vi "Read Instr XML File.vi"(0 "XML File Name":string, 5 "error in (no error)":errorcluster) -> (10 "Instr 1 Resource Str":string, 11 "Instr 4 Class Path":path, 12 "Instr 1 Class Path":path, 13 "Instr 4 Resource Str":string, 14 "Instr 2 Resource Str":string, 15 "Instr 2 Class Path":path, 16 "Instr 3 Resource Str":string, 17 "Instr 3 Class Path":path, 19 "error IO":errorcluster)   [LabVIEW 2010]
doc: "Reads an XML file with the DSSP module and hardware resource name information."
uses:
  <vilib>/Utility/xml.llb/Read From XML File(array).vi
panel:
  out "Instr 4 type":string
  out "Instr 3 type":string
  out "Instr 2 type":string
  out "Instr 1 type":string
  out "XML File Path Out":path
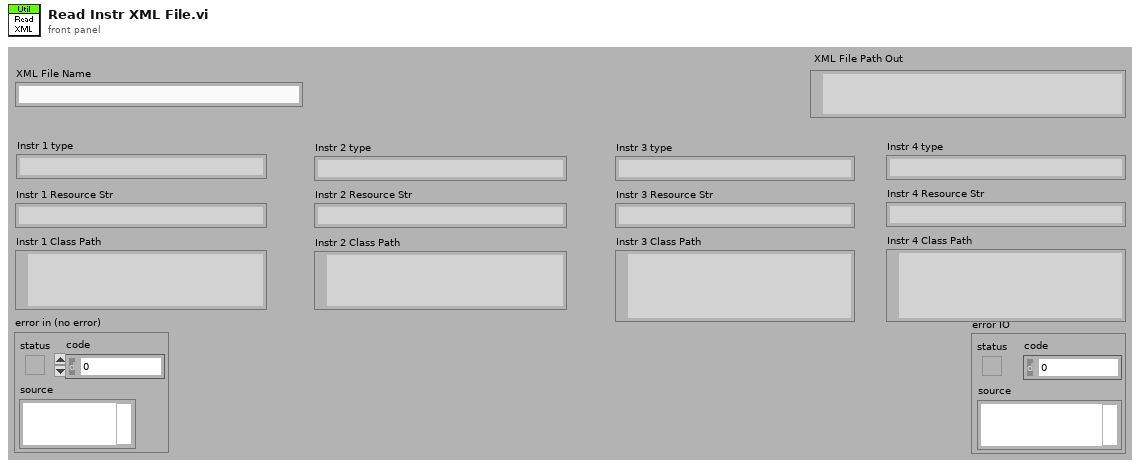
[diagram p1: front panel]
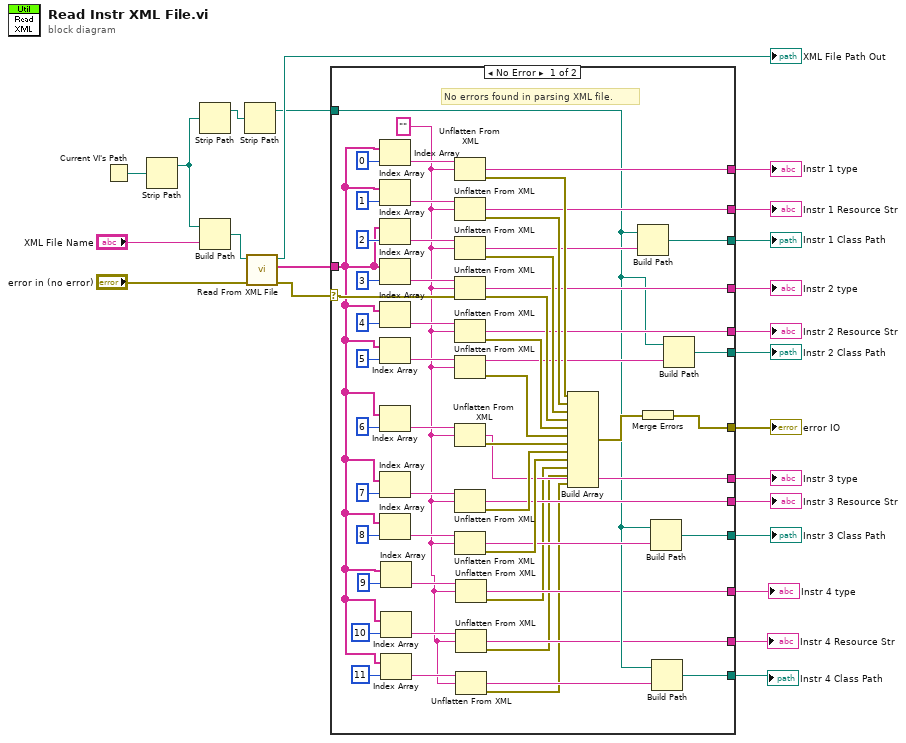
[diagram p0: block diagram]
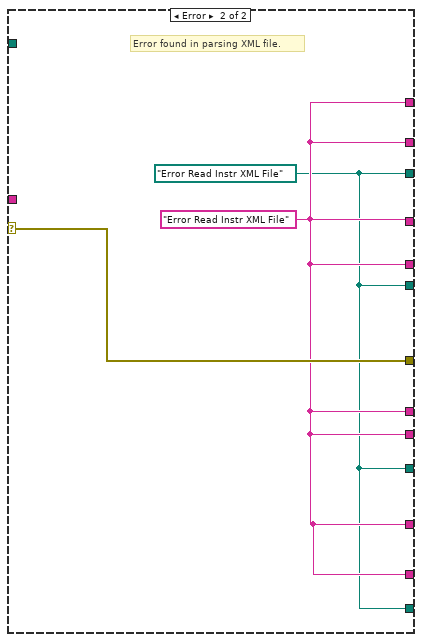
[diagram p2: hidden frame]
diagram:
  n1 = Current VI's Path() -> (path=w9:path)
  n2 = Strip Path(path=w9) -> (stripped path=w7:path)  [unwired: 1 out]
  n3 = Strip Path(path=w7) -> (stripped path=w5:path)  [unwired: 1 out]
  n4 = Build Path(base path=w7, name or relative path="XML File Name") -> (appended path=w8:path)
  n5 = Strip Path(path=w5) -> (stripped path=w4:path)  [unwired: 1 out]
  n6 = call-poly <vilib>:"Read From XML File.vi"("error in (no error)"="error in (no error)", "XML File Path"=w8) -> ("error out"=w21:errorcluster, "XML Elements"=w22:string[], "XML File Path(duplicate)"=→"XML File Path Out":path)  [unwired: 7 out]
  n7 = case shown="No Error" w21 {
    selector: w21 -> [w47 w84]
    tunnel: w22 -> [w36 _]
    tunnel: [w68 w84] -> w13
    tunnel: [w50 w83] -> w20
    tunnel: [w44 w82] -> w19
    tunnel: [w52 w83] -> w18
    tunnel: [w42 w82] -> w17
    tunnel: [w51 w83] -> w16
    tunnel: [w40 w82] -> w15
    tunnel: [w49 w83] -> w12
    tunnel: [w48 w83] -> w11
    tunnel: [w46 w83] -> w10
    tunnel: w4 -> [w31 _]
    tunnel: [w29 w82] -> w3
    tunnel: [w28 w83] -> w2
    tunnel: [w27 w83] -> w1
    frame No Error {
      w32 = ""
      # "No errors found in parsing XML file."
      n8 = Index Array(array=w36, index=0) -> (element=w77:string)
      n9 = Index Array(array=w36, index=1) -> (element=w76:string)
      n10 = Index Array(array=w36, index=2) -> (element=w75:string)
      n11 = Index Array(array=w36, index=3) -> (element=w74:string)
      n12 = Index Array(array=w36, index=4) -> (element=w62:string)
      n13 = Index Array(array=w36, index=5) -> (element=w61:string)
      n14 = Index Array(array=w36, index=6) -> (element=w60:string)
      n15 = Index Array(array=w36, index=7) -> (element=w59:string)
      n16 = Index Array(array=w36, index=8) -> (element=w58:string)
      n17 = Index Array(array=w36, index=9) -> (element=w33:string)
      n18 = Index Array(array=w36, index=10) -> (element=w35:string)
      n19 = Index Array(array=w36, index=11) -> (element=w34:string)
      n20 = Unflatten From XML(xml string=w77, type=w32) -> (value=w50:string, error out=w73:errorcluster)  [unwired: 1 in]
      n21 = Unflatten From XML(xml string=w76, type=w32) -> (value=w49:string, error out=w72:errorcluster)  [unwired: 1 in]
      n22 = Unflatten From XML(xml string=w75, type=w32) -> (value=w45:string, error out=w71:errorcluster)  [unwired: 1 in]
      n23 = Unflatten From XML(xml string=w74, type=w32, error in (no error)=w47) -> (value=w52:string, error out=w70:errorcluster)
      n24 = Unflatten From XML(xml string=w62, type=w32) -> (value=w48:string, error out=w57:errorcluster)  [unwired: 1 in]
      n25 = Unflatten From XML(xml string=w61, type=w32) -> (value=w41:string, error out=w56:errorcluster)  [unwired: 1 in]
      n26 = Unflatten From XML(xml string=w60, type=w32) -> (value=w51:string, error out=w55:errorcluster)  [unwired: 1 in]
      n27 = Unflatten From XML(xml string=w59, type=w32) -> (value=w46:string, error out=w54:errorcluster)  [unwired: 1 in]
      n28 = Unflatten From XML(xml string=w58, type=w32) -> (value=w43:string, error out=w53:errorcluster)  [unwired: 1 in]
      n29 = Unflatten From XML(xml string=w33, type=w32) -> (value=w27:string, error out=w26:errorcluster)  [unwired: 1 in]
      n30 = Unflatten From XML(xml string=w35, type=w32) -> (value=w28:string, error out=w25:errorcluster)  [unwired: 1 in]
      n31 = Unflatten From XML(xml string=w34, type=w32) -> (value=w30:string, error out=w24:errorcluster)  [unwired: 1 in]
      n32 = Build Array(w73, w72, w71, w70, w57, w56, w55, w54, w53, w26, w25, w24) -> (w69:errorcluster[])
      n33 = Build Path(base path=w31, name or relative path=w45) -> (appended path=w44:path)
      n34 = Merge Errors(w69) -> (w68:errorcluster)
      n35 = Build Path(base path=w31, name or relative path=w43) -> (appended path=w40:path)
      n36 = Build Path(base path=w31, name or relative path=w30) -> (appended path=w29:path)
      n37 = Build Path(base path=w31, name or relative path=w41) -> (appended path=w42:path)
    }
    frame Error {
      w82 = path "Error Read Instr XML File" ("XML File Path Out 2")
      w83 = "Error Read Instr XML File"
      # "Error found in parsing XML file."
    }
  }
  "Instr 1 type" <- w20
  "Instr 1 Class Path" <- w19
  "Instr 2 type" <- w18
  "Instr 2 Class Path" <- w17
  "Instr 3 type" <- w16
  "Instr 3 Class Path" <- w15
  "error IO" <- w13
  "Instr 1 Resource Str" <- w12
  "Instr 2 Resource Str" <- w11
  "Instr 3 Resource Str" <- w10
  "Instr 4 type" <- w1
  "Instr 4 Class Path" <- w3
  "Instr 4 Resource Str" <- w2
